vi "Write Motor PID Gains.vi"(8 "error in (no error)":errorcluster, 10 "motor PID gains":T1={"proportional gain (Kc)"=0.25, "integral gain (Kc*Ts/Ti)"=0.3984375, "derivative gain (Kc*Td/Ts)"=0.01171875}, 11 "starter kit host in":refnum<class "NI_Robotics_Starter Kit Host_FPGA_1.0.lvclass">) -> (0 "error out":errorcluster, 3 "starter kit host out":refnum<class "NI_Robotics_Starter Kit Host_FPGA_1.0.lvclass">)   [LabVIEW 2017, in "NI_Robotics_Starter Kit Host_FPGA_1.0.lvclass"]
uses:
  <vilib>/robotics/Starter Kit/1.0/FPGA Host Interface/NI_Robotics_Starter Kit Host_FPGA_1.0.lvclass
  <vilib>/robotics/Starter Kit/1.0/FPGA Host Interface/NI_Robotics_Starter Kit Host_FPGA_1.0.lvclass/NI_Robotics_Starter Kit Host_FPGA_1.0.ctl
  <vilib>/rvi/errors/niLvFpgaAdjustHostInterfaceError.vi
  <vilib>/Utility/error.llb/Error Cluster From Error Code.vi
  <vilib>/robotics/Starter Kit/1.0/FPGA Host Interface/FPGA Refnum.ctl
  <vilib>/rvi/interface/nirviReadWriteControl/nirviReadWriteControl.xnode
  NiFpgaLv.dll
  <vilib>/rvi/interface/Simulation/niFpgaSimulationCallBeginRW.vi
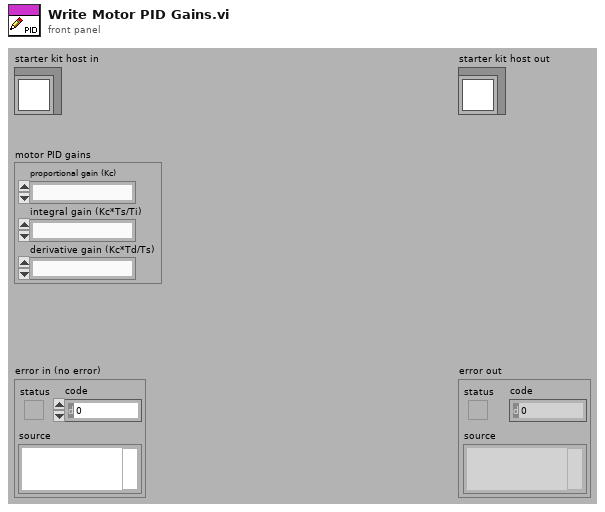
[diagram p1: front panel]
types:
  T1 = cluster{"proportional gain (Kc)":fxp<+/-,16,8>, "integral gain (Kc*Ts/Ti)":fxp<+/-,16,8>, "derivative gain (Kc*Td/Ts)":fxp<+/-,16,8>}
  T2 = typedef "NI_Robotics_Starter Kit Host_FPGA_1.0.lvclass/FPGA Refnum.ctl" = refnum<k20>
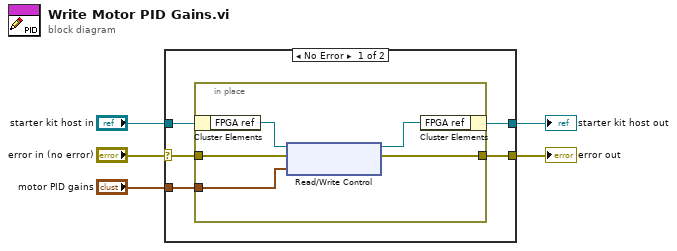
[diagram p0: block diagram]
diagram:
  n1 = case shown="No Error" "error in (no error)" {
    selector: "error in (no error)" -> [w8 w17]
    tunnel: "starter kit host in" -> [w10 w16]
    tunnel: [w7 w17] -> w3
    tunnel: [w6 w16] -> w2
    tunnel: "motor PID gains" -> [w9 _]
    frame No Error {
      n2 = in-place {
        in-place-border: w9 -> [w14]
        in-place-border: w8 -> [w13]
        in-place-border: [w12] -> w7
        n3 = in-place-cluster #1(w10) -> ("FPGA ref"=w15:T2)
        n4 = xnode "Read/Write Control"("FPGA VI Reference In"=w15, "error in"=w13, "motor PID gains"=w14) -> ("FPGA VI Reference Out"=w11:T2, "error out"=w12:errorcluster)
        n5 = in-place-cluster #1("FPGA ref"=w11) -> (w6:refnum<class "NI_Robotics_Starter Kit Host_FPGA_1.0.lvclass">)
      }
    }
    frame Error {
    }
  }
  "error out" <- w3
  "starter kit host out" <- w2
